vi "Motion_Read Error Codes.vi"(8 "error in (no error)":errorcluster, 11 "TCP Connection Refnum in":refnum<k5>) -> (0 "error out":errorcluster, 1 "Controller Alarm":u32, 2 "Errors":cluster{"Error ID":u16, "Error String":string}[](array[cluster]), 3 "TCP Connection Refnum (dup)":refnum<k5>)   [LabVIEW 2010]
uses:
  <vilib>/NI Modbus.llb/MB Ethernet Master Query Read Input Registers (poly).vi
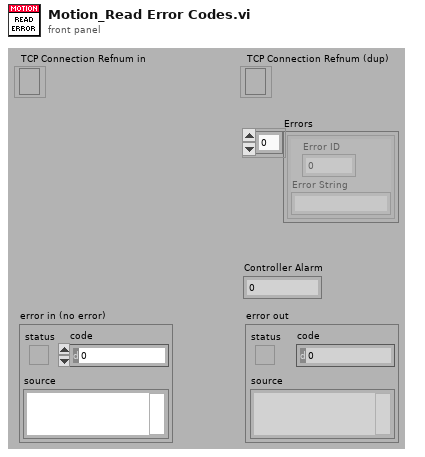
[diagram p1: front panel]
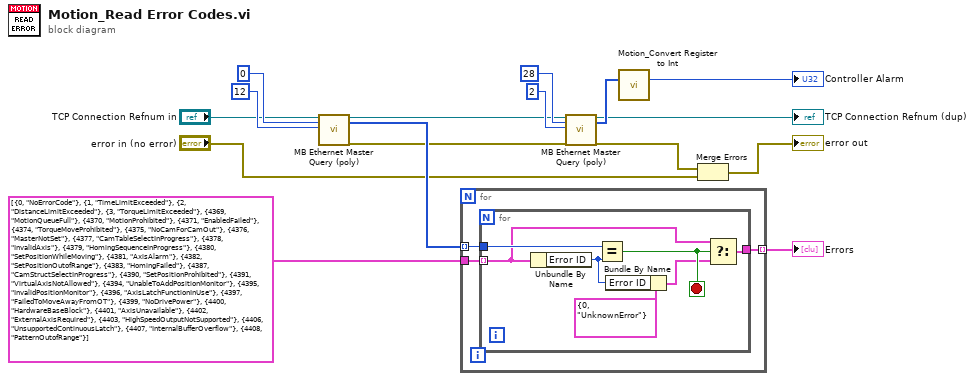
[diagram p0: block diagram]
diagram:
  n1 = call-poly <vilib>:"MB Ethernet Master Query (poly).vi"("TCP Connection Refnum in"="TCP Connection Refnum in", "Starting Address"=u16 0, "Quantity"=u16 12 ("Quantity 2")) -> ("TCP Connection Refnum (dup)"=w5:refnum<k5>, "Input Registers"=w12:u16[], "error out"=w6:errorcluster)  [unwired: 13 in, 1 out]
  n2 = for {
    tunnel: cluster{"Error ID":u16, "Error String":string}[] [{"Error ID"=0, "Error String"="NoErrorCode"}, {"Error ID"=1, "Error String"="TimeLimitExceeded"}, {"Error ID"=2, "Error String"="DistanceLimitExceeded"}, {"Error ID"=3, "Error String"="TorqueLimitExceeded"}, {"Error ID"=4369, "Error String"="MotionQueueFull"}, {"Error ID"=4370, "Error String"="MotionProhibited"}, {"Error ID"=4371, "Error String"="EnabledFailed"}, {"Error ID"=4374, "Error String"="TorqueMoveProhibited"}, {"Error ID"=4375, "Error String"="NoCamForCamOut"}, {"Error ID"=4376, "Error String"="MasterNotSet"}, {"Error ID"=4377, "Error String"="CamTableSelectInProgress"}, {"Error ID"=4378, "Error String"="InvalidAxis"}, {"Error ID"=4379, "Error String"="HomingSequenceInProgress"}, {"Error ID"=4380, "Error String"="SetPositionWhileMoving"}, {"Error ID"=4381, "Error String"="AxisAlarm"}, {"Error ID"=4382, "Error String"="SetPositionOutofRange"}, {"Error ID"=4383, "Error String"="HomingFailed"}, {"Error ID"=4387, "Error String"="CamStructSelectInProgress"}, {"Error ID"=4390, "Error String"="SetPositionProhibited"}, {"Error ID"=4391, "Error String"="VirtualAxisNotAllowed"}, {"Error ID"=4394, "Error String"="UnableToAddPositionMonitor"}, {"Error ID"=4395, "Error String"="InvalidPositionMonitor"}, {"Error ID"=4396, "Error String"="AxisLatchFunctionInUse"}, {"Error ID"=4397, "Error String"="FailedToMoveAwayFromOT"}, {"Error ID"=4399, "Error String"="NoDrivePower"}, {"Error ID"=4400, "Error String"="HardwareBaseBlock"}, {"Error ID"=4401, "Error String"="AxisUnavailable"}, {"Error ID"=4402, "Error String"="ExternalAxisRequired"}, {"Error ID"=4403, "Error String"="HighSpeedOutputNotSupported"}, {"Error ID"=4406, "Error String"="UnsupportedContinuousLatch"}, {"Error ID"=4407, "Error String"="InternalBufferOverflow"}, {"Error ID"=4408, "Error String"="PatternOutofRange"}] ("Error ID") -> [w19]
    tunnel: w12 -> [w18] mode=indexing
    tunnel: [w17] -> w11 mode=indexing
    n3 = for {
      tunnel: w19 -> [w24] mode=indexing
      tunnel: w18 -> [w26]
      tunnel: [w20] -> w17
      stop <- w25 stop-if-true
      n4 = Unbundle By Name(w24) -> ("Error ID"=w22:u16)
      n5 = Equal?(x=w26, y=w22) -> (x = y?=w25:bool)
      n6 = Bundle By Name(cluster=cluster{"Error ID":u16, "Error String":string} {"Error ID"=0, "Error String"="UnknownError"}, "Error ID"=w22) -> (w21:cluster{"Error ID":u16, "Error String":string})
      n7 = Select(t=w24, s=w25, f=w21) -> (s? t:f=w20:cluster{"Error ID":u16, "Error String":string})
    }
  }
  "Errors" <- w11
  n8 = call-poly <vilib>:"MB Ethernet Master Query (poly).vi"("TCP Connection Refnum in"=w5, "Starting Address"=u16 28, "Quantity"=u16 2, "error in"=w6) -> ("TCP Connection Refnum (dup)"=→"TCP Connection Refnum (dup)":refnum<k5>, "Input Registers"=w8:u16[], "error out"=w2:errorcluster)  [unwired: 12 in, 1 out]
  n9 = call "Motion_Convert Register to Int.vi"("Register array"=w8) -> ("Int"=→"Controller Alarm":u32)  [unwired: 14 in]
  n10 = Merge Errors(w2, "error in (no error)") -> (→"error out":errorcluster)
